vi "Set Decoration Tag.vi"(8 "error in (no error)":errorcluster, 11 "VI Refnum":refnum<vi>) -> (0 "error out":errorcluster)   [LabVIEW 2017]
uses:
  <vilib>/UserTags/UserTags.lvlib
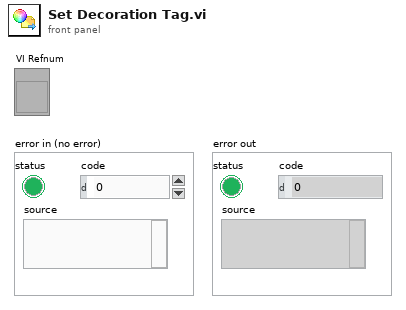
[diagram p1: front panel]
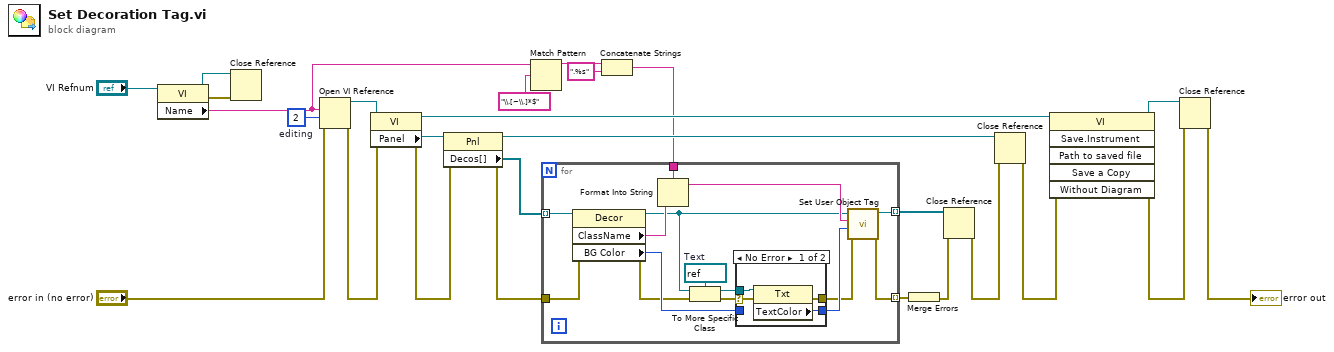
[diagram p0: block diagram]
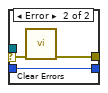
[diagram p2: hidden frame]
diagram:
  w26 = 2  # editing
  n1 = property class="VI"(reference="VI Refnum") -> (reference out=w22:refnum<vi>, error out=w23:errorcluster, "Name"=w5:string)  [unwired: 1 in]
  n2 = Close Reference(reference=w22, error in (no error)=w23) -> ()  [unwired: 1 out]
  n3 = Open VI Reference(vi path=w5, options=w26, error in (no error)="error in (no error)") -> (vi reference=w25:refnum<vi>, error out=w19:errorcluster)  [unwired: 3 in]
  n4 = property class="VI"(reference=w25, error in=w19) -> (reference out=w20:refnum<vi>, error out=w18:errorcluster, "Panel"=w24:refnum<vi>)
  n5 = property class="Pnl"(reference=w24, error in=w18) -> (reference out=w13:refnum<vi>, error out=w16:errorcluster, "Decos[]"=w21:refnum<vi>[])
  n6 = Match Pattern(string=w5, regular expression="\\.[~\\.]*$") -> (before substring=w3:string)  [unwired: 4 out]
  n7 = Concatenate Strings(w3, ".%s" ("string")) -> (w1:string)
  n8 = for {
    tunnel: w21 -> [w41] mode=indexing
    tunnel: w1 -> [w40]
    tunnel: [w30] -> w17 mode=indexing
    tunnel: w16 -> [w28]
    tunnel: [w27] -> w14 mode=indexing
    w36 = refnum<vi> refnum  # Text
    n9 = property class="Decor"(reference=w41, error in=w28) -> (reference out=w37:refnum<vi>, error out=w29:errorcluster, "ClassName"=w39:string, "BG Color"=w33:u32)
    n10 = Format Into String(format string=w40, w39) -> (resulting string=w38:string)  [unwired: 2 in, 1 out]
    n11 = To More Specific Class(target class=w36, reference=w37, error in=w29) -> (specific class reference=w35:refnum<vi>, error out=w34:errorcluster)
    n12 = case shown="No Error" w34 {
      selector: w34 -> [w42 w47]
      tunnel: w35 -> [w45 _]
      tunnel: w33 -> [_ w48]
      tunnel: [w44 w48] -> w32
      tunnel: [w43 w46] -> w31
      frame No Error {
        n13 = property class="Txt"(reference=w45, error in=w42) -> (error out=w43:errorcluster, "TextColor"=w44:u32)  [unwired: 1 out]
      }
      frame Error {
        n14 = call <vilib>:"Clear Errors.vi"("error in (no error)"=w47) -> ("error out"=w46:errorcluster)  [unwired: 5 in, 1 out]
      }
    }
    n15 = call <vilib>:"Set User Object Tag.vi"("error in (no error)"=w31, "Value"=w32, "Tag Name"=w38, "Generic Refnum"=w37) -> ("error out"=w30:errorcluster, "dup Generic Refnum"=w27:refnum<vi>)  [unwired: 5 in, 1 out]
  }
  n16 = Merge Errors(w17) -> (w11:errorcluster)
  n17 = Close Reference(reference=w14, error in (no error)=w11) -> (error out=w12:errorcluster)
  n18 = Close Reference(reference=w13, error in (no error)=w12) -> (error out=w10:errorcluster)
  n19 = invoke class="VI" method="Save.Instrument"(reference=w20, error in=w10) -> (reference out=w9:refnum<vi>, error out=w8:errorcluster)  [unwired: 4 in, 4 out]
  n20 = Close Reference(reference=w9, error in (no error)=w8) -> (error out=→"error out":errorcluster)
